vi "纳清电导率_所有参数读取.vi"(8 "error in (no error)":errorcluster caption="错误输入（无错误）", 11 "MB session in":refnum<class "MB_Master.lvclass">) -> (0 "error out":errorcluster caption="错误输出", 2 "输出值":T1 {"波特率" items=["4800", "9600", "19200", "38400", "57600", "115200"]}, 3 "MB session out":refnum<class "MB_Master.lvclass">)   [LabVIEW 2016, in "斯坦道多参数.lvlib"]
uses:
  <vilib>/Plasmionique/MB Master/MB_Master/MB_Master.lvclass
  <vilib>/Plasmionique/MB Master/MB Master.lvlib
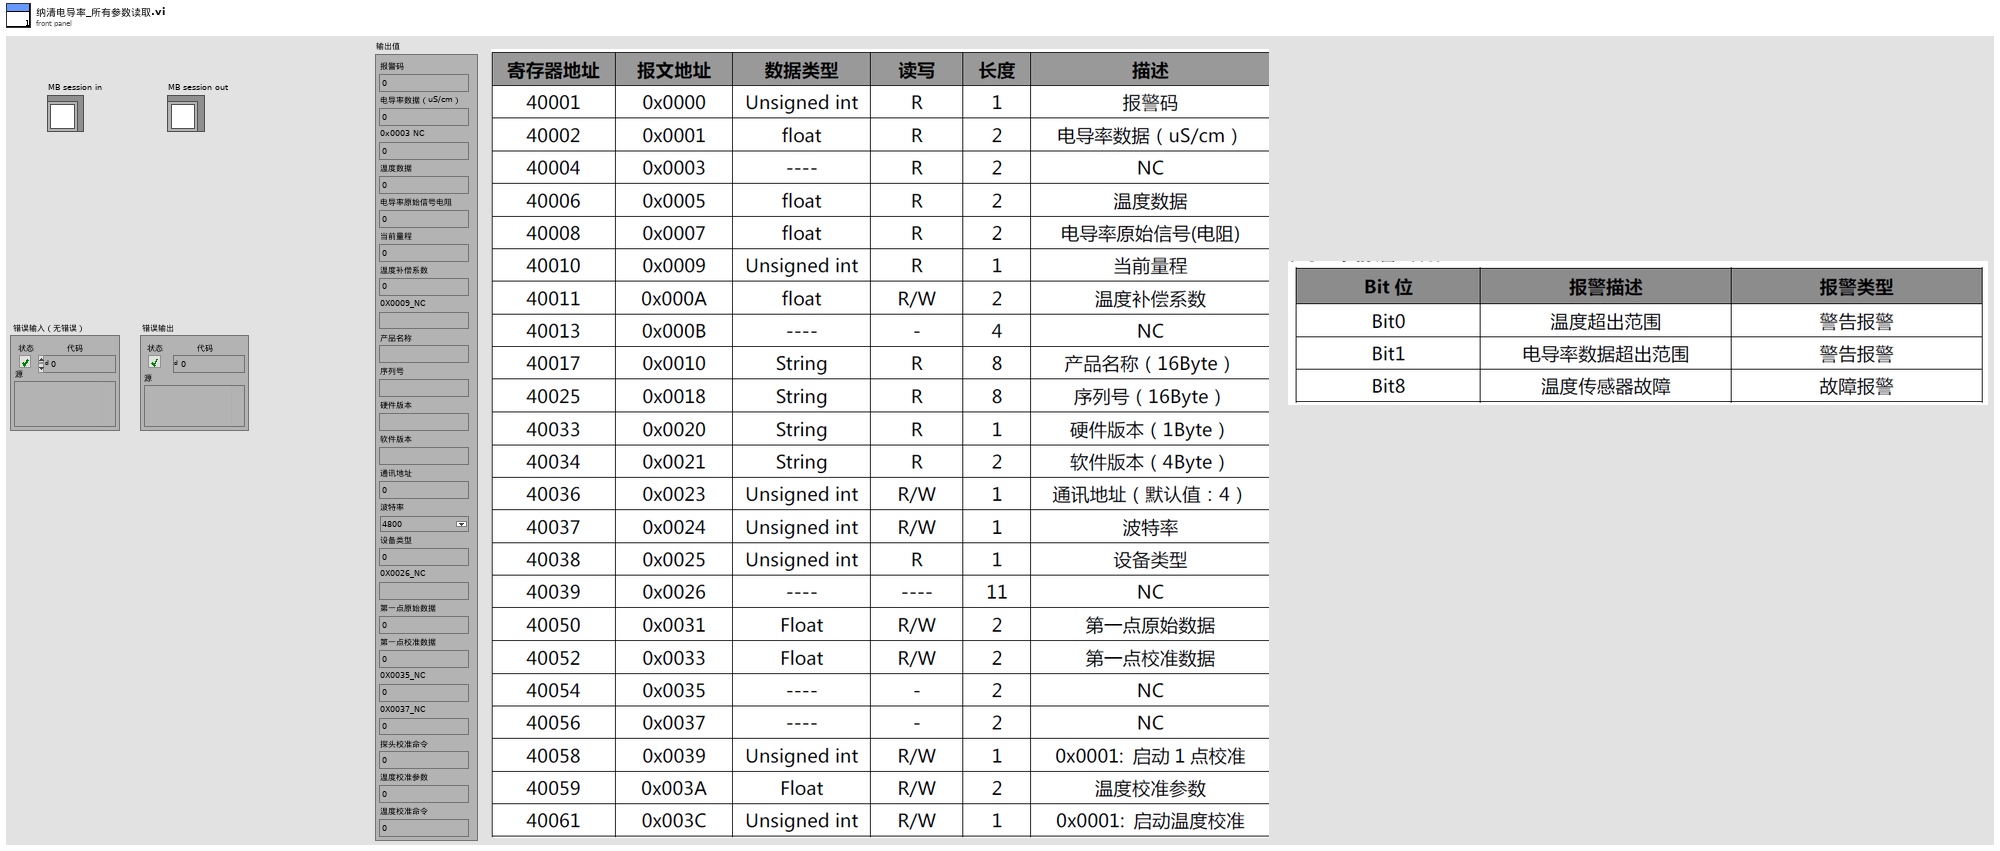
[diagram p1: front panel]
types:
  T1 = cluster{"报警码":u16, "电导率数据（uS/cm）":sgl, "0x0003 NC":sgl, "温度数据":sgl, "电导率原始信号电阻":sgl, "当前量程":u16, "温度补偿系数":sgl, "0X0009_NC":string, "产品名称":string, "序列号":string, "硬件版本":string, "软件版本":string, "通讯地址":u16, "波特率":u16, "设备类型":u16, "0X0026_NC":string, "第一点原始数据":sgl, "第一点校准数据":sgl, "0X0035_NC":sgl, "0X0037_NC":sgl, "探头校准命令":u16, "温度校准参数":sgl, "温度校准命令":u16}
  T2 = cluster{"pH":u32, "DO":u32, "Cond":u32, "Turb":u32, "叶绿素a":u32, "藻密度":u32, "ORP":u32}
  T3 = cluster{u16, "mode":dbl, "数值":sgl, "数值":sgl, "数值":sgl, u16, "数值":sgl, "类型":string, "类型":string, "类型":string, "类型":string, "类型":string, u16, u16, u16, "类型":string, "数值":sgl, "数值":sgl, "数值":sgl, "数值":sgl, u16, "数值":sgl, u16}
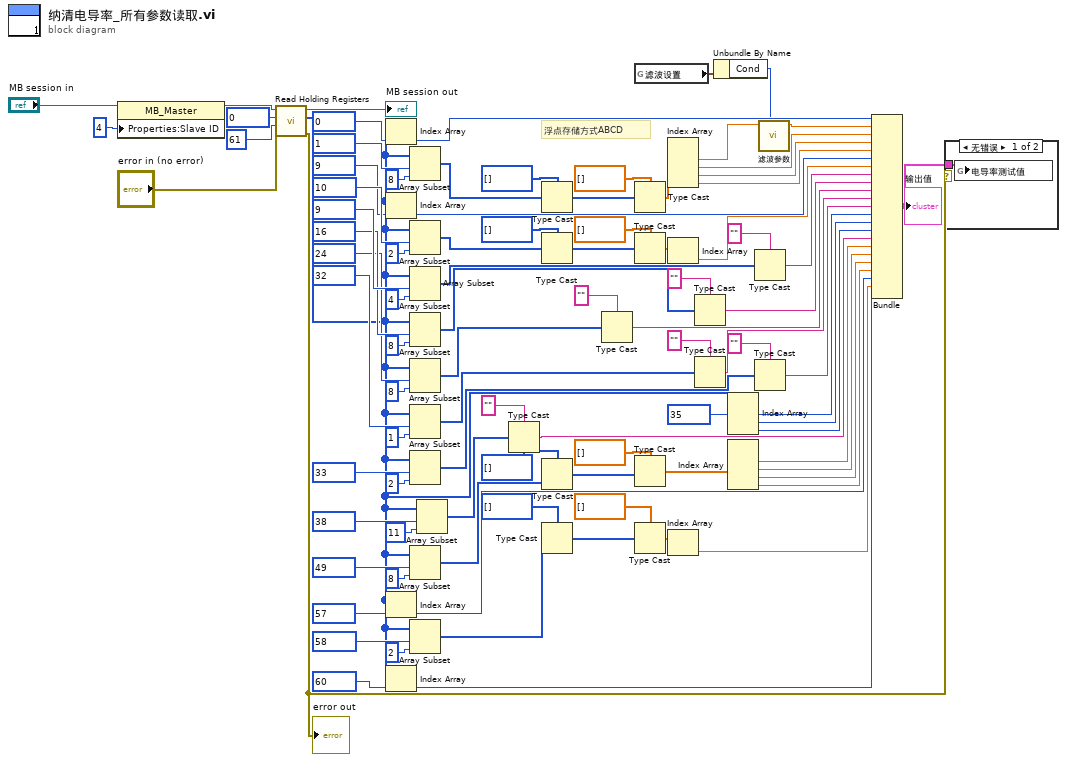
[diagram p0: block diagram]
diagram:
  # "浮点存储方式ABCD"
  n1 = property class="MB_Master"(reference="MB session in", "Properties:Slave ID"=u8 4 ("Slave ID")) -> (reference out=w83:refnum<class "MB_Master.lvclass">)  [unwired: 1 in, 1 out]
  n2 = call <vilib>:"Read Holding Registers.vi"("error in (no error)"="error in (no error)", "quantity"=u16 61, "starting address"=u16 0, "MB session in"=w83) -> ("error out"=w25:errorcluster, "Registers"=w6:u16[], "MB session out"=→"MB session out":refnum<class "MB_Master.lvclass">)  [unwired: 5 in]
  "error out" <- w25
  n3 = Index Array(array=w6, index=u16 0 ("starting address")) -> (element=w91:u16)
  n4 = Index Array(array=w6, index=u16 9 ("starting address")) -> (element=w5:u16)
  n5 = Index Array(array=w6, index=u16 57 ("starting address")) -> (element=w29:u16)
  n6 = Index Array(array=w6, index=u16 60 ("starting address")) -> (element=w26:u16)
  n7 = Array Subset(array=w6, index=u16 1 ("starting address"), length=8 ("长度")) -> (w87:u16[])
  n8 = Array Subset(array=w6, index=u16 10 ("starting address"), length=2 ("长度")) -> (w9:u16[])
  n9 = Array Subset(array=w6, index=u16 9 ("starting address"), length=4 ("长度")) -> (w77:u16[])
  n10 = Array Subset(array=w6, index=u16 16 ("starting address"), length=8 ("长度")) -> (w73:u16[])
  n11 = Array Subset(array=w6, index=u16 24 ("starting address"), length=8 ("长度")) -> (w67:u16[])
  n12 = Array Subset(array=w6, index=u16 32 ("starting address"), length=1 ("长度")) -> (w63:u16[])
  n13 = Array Subset(array=w6, index=u16 33 ("starting address"), length=2 ("长度")) -> (w57:u16[])
  n14 = Array Subset(array=w6, index=u16 49 ("starting address"), length=8 ("长度")) -> (w44:u16[])
  n15 = Array Subset(array=w6, index=u16 58 ("starting address"), length=2 ("长度")) -> (w32:u16[])
  n16 = Array Subset(array=w6, index=u16 38 ("starting address"), length=11 ("长度")) -> (w47:u16[])
  n17 = Type Cast(type="" ("类型"), x=w47) -> (*(type *) &x=w46:string)
  n18 = Type Cast(type=u32[] [] ("数组 2"), x=w87) -> (*(type *) &x=w24:u32[])
  n19 = Type Cast(type=u32[] [] ("数组 2"), x=w9) -> (*(type *) &x=w13:u32[])
  n20 = Type Cast(type=u32[] [] ("数组 2"), x=w44) -> (*(type *) &x=w42:u32[])
  n21 = Type Cast(type=u32[] [] ("数组 2"), x=w32) -> (*(type *) &x=w34:u32[])
  n22 = Type Cast(type="" ("类型"), x=w67) -> (*(type *) &x=w65:string)
  n23 = global read "断电保存变量.vi" "滤波设置"() -> (w2:T2)
  n24 = Type Cast(type=sgl[] [] ("数组 2"), x=w24) -> (*(type *) &x=w86:sgl[])
  n25 = Type Cast(type=sgl[] [] ("数组 2"), x=w13) -> (*(type *) &x=w12:sgl[])
  n26 = Type Cast(type=sgl[] [] ("数组 2"), x=w42) -> (*(type *) &x=w39:sgl[])
  n27 = Type Cast(type=sgl[] [] ("数组 2"), x=w34) -> (*(type *) &x=w37:sgl[])
  n28 = Index Array(array=w86) -> (element #1=w4:sgl, element #2=w81:sgl, element #3=w21:sgl, element #4=w20:sgl)  [unwired: 4 in]
  n29 = Index Array(array=w12) -> (element=w8:sgl)  [unwired: 1 in]
  n30 = Index Array(array=w37) -> (element=w28:sgl)  [unwired: 1 in]
  n31 = Type Cast(type="" ("类型"), x=w73) -> (*(type *) &x=w70:string)
  n32 = Type Cast(type="" ("类型"), x=w63) -> (*(type *) &x=w60:string)
  n33 = Unbundle By Name(w2) -> ("Cond"=w1:u32)
  n34 = Index Array(array=w6, index #1=u16 35 ("starting address")) -> (element #1=w53:u16, element #2=w52:u16, element #3=w51:u16)  [unwired: 2 in]
  n35 = Index Array(array=w39) -> (element #1=w38:sgl, element #2=w19:sgl, element #3=w18:sgl, element #4=w17:sgl)  [unwired: 4 in]
  n36 = Type Cast(type="" ("类型"), x=w77) -> (*(type *) &x=w75:string)
  n37 = Type Cast(type="" ("类型"), x=w57) -> (*(type *) &x=w55:string)
  n38 = call "滤波参数.vi"("滤波次数"=w1, "x"=w4) -> ("mode"=w3:dbl)  [unwired: 9 in]
  n39 = Bundle(w91, "mode"=w3, "数值"=w81, "数值"=w21, "数值"=w20, w5, "数值"=w8, "类型"=w75, "类型"=w70, "类型"=w65, "类型"=w60, "类型"=w55, w53, w52, w51, "类型"=w46, "数值"=w38, "数值"=w19, "数值"=w18, "数值"=w17, w29, "数值"=w28, w26) -> (w16:T3)  [unwired: 1 in]
  "输出值" <- w16
  n40 = case shown="无错误" w25 {
    tunnel: w16 -> [w94 _]
    frame No Error {
      n41 = global write "纳清过程全局变量.vi" "电导率测试值"(w94) -> ()
    }
    frame Error {
    }
  }
